vi "saveTimeSeries_I.vi"(0 "422nm":dbl, 1 "file path (dialog if empty)":path, 2 "save?":bool, 11 "Error In":errorcluster) -> (15 "Error Out":errorcluster)   [LabVIEW 2011]
uses:
  <vilib>/Utility/file.llb/Write To Spreadsheet File (string).vi
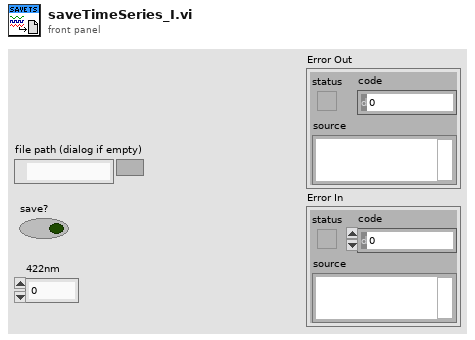
[diagram p1: front panel]
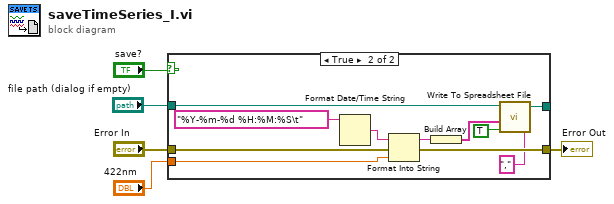
[diagram p0: block diagram]
diagram:
  n1 = case shown="True" "save?" {
    tunnel: "422nm" -> [_ w18]
    tunnel: "file path (dialog if empty)" -> [w7 w17]
    tunnel: [w7 w16] -> _
    tunnel: "Error In" -> [w6 w10]
    tunnel: [w6 w9] -> w3
    frame False {
    }
    frame True {
      n2 = Format Date/Time String(time format string (%c)="%Y-%m-%d %H:%M:%S\t") -> (date/time string=w14:string)  [unwired: 2 in]
      n3 = Format Into String(initial string=w14, error in=w10, w18) -> (resulting string=w12:string, error out=w9:errorcluster)  [unwired: 1 in]
      n4 = Build Array(w12) -> (w11:string[])
      n5 = call-poly <vilib>:"Write To Spreadsheet File.vi"("delimiter (\\t)"="," ("delimiter (\\t)"), "append to file? (new file:F)"=TRUE, "1D data"=w11, "file path (dialog if empty)"=w17) -> ("new file path (Not A Path if cancelled)"=w16:path)  [unwired: 4 in]
    }
  }
  "Error Out" <- w3
